vi "FTW-Actor.vi"(0 "DD Actor Template-Core In":refnum<class "DD Actor Template-Core.lvclass">, 5 "FTW Actor Instance Configuration":string="{\n  \"Identity\": \"ActorName\",\n  \"InboxAddress\": \"inproc://*\",\n  \"LoggerAddress\": \"\",\n  \"My Data\": false,\n  \"Publisher URI\": \"inproc://*\",\n  \"Subscriber URIs\": \"\",\n  \"Refresh Period\": 2\n}", 11 "ErrorIn":errorcluster) -> (15 "Error":errorcluster)   [LabVIEW 2018, in "DD Actor Template-Core.lvclass"]
uses:
  DD Actor Template-Core.lvclass
  C:/Jobs/Featherweight/featherweight-2018/source/actor/Instance/FTW-ActorInstance.lvclass
  DD Actor Template-Core.lvclass/DD Actor Template-Core.ctl
  source/actor/Instance/FTW-ActorInstance.lvclass/FTW-ActorInstance.ctl
  b528c082-742f-4d18-8b03-c390aae6fd68.vi
  b528c082-742f-4d18-8b03-c390aae6fd68.vi/37bc4ba9-e295-41d8-9da2-04944fffb029.vi
  source/container/FTW-Container-FromVariant.vi
  source/container/FTW-Container-New-FromContainer.vi
  source/JSON/FTW-JSON-SerializeAndDestroy.vi
  source/actor/JobSequencer/FTW-SEQ-Current.vi
  source/actor/Message/Base/FTW-Message.lvclass
  source/actor/Connector/FTW-ActorConnector.lvclass
  source/actor/Instance/FTW-ActorInstance.lvclass
  source/actor/Message/Request/FTW-Message-IncomingRequest.lvclass
  source/actor/Publisher/FTW-Publisher.lvclass
  source/actor/Subscriber/FTW-Subscriber.lvclass
panel:
  # "#TODO\nhide controls for a GUI"
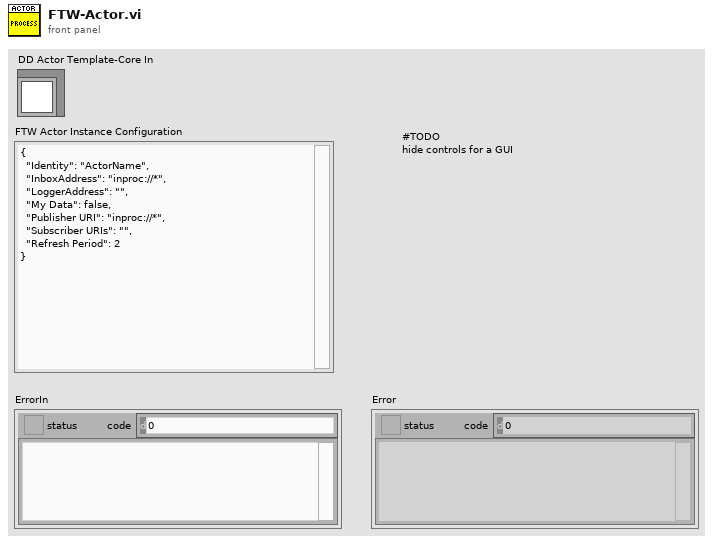
[diagram p1: front panel]
types:
  T1 = cluster{"Incoming Requests":refnum<event-registration>, "Local Messages":refnum<event-registration>, "Subscriber Registration":refnum<event-registration>}
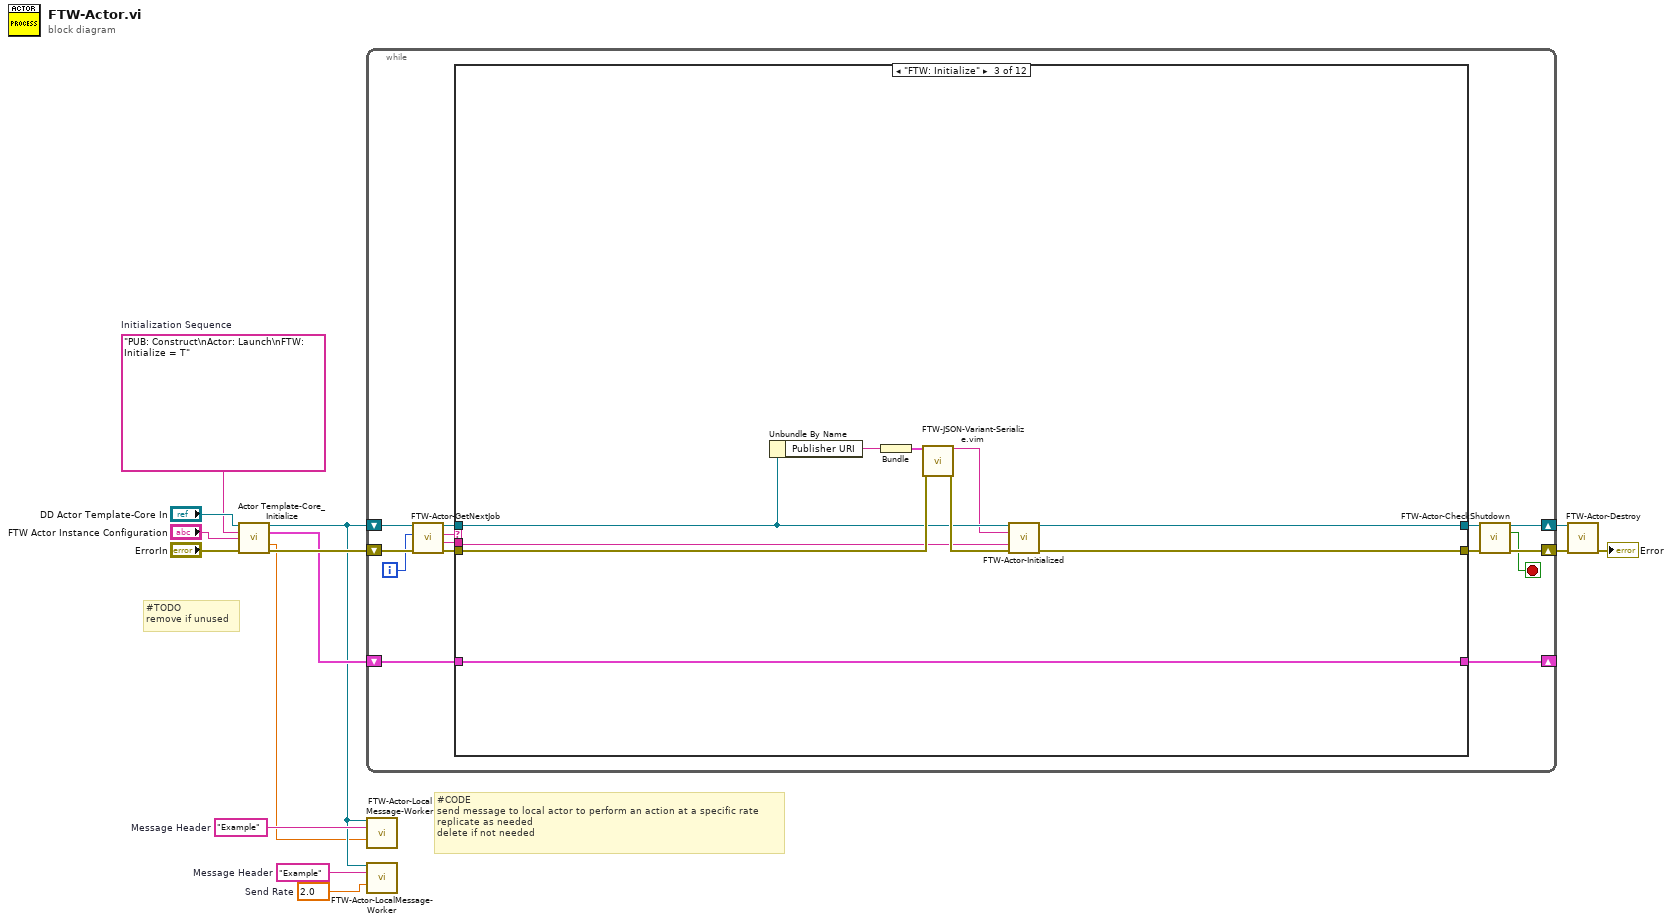
[diagram p0: block diagram]
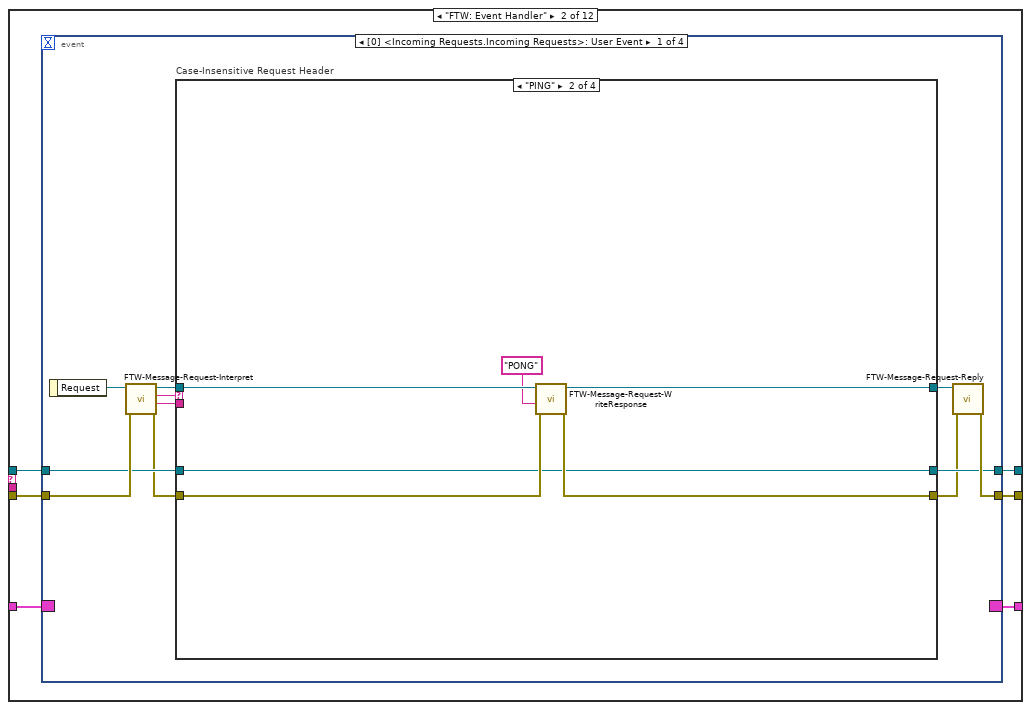
[diagram p3: hidden frame]
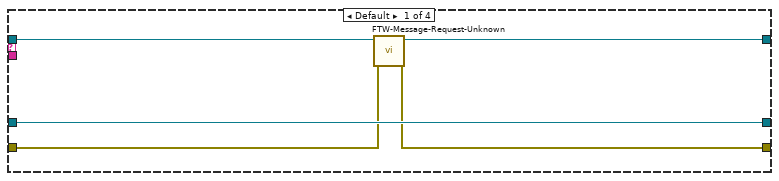
[diagram p4: hidden frame]
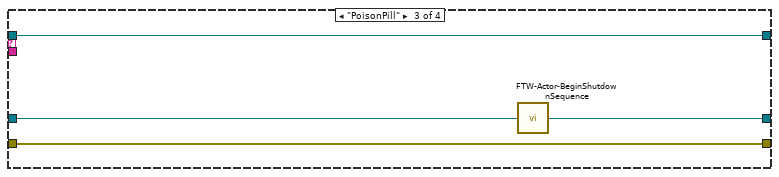
[diagram p5: hidden frame]
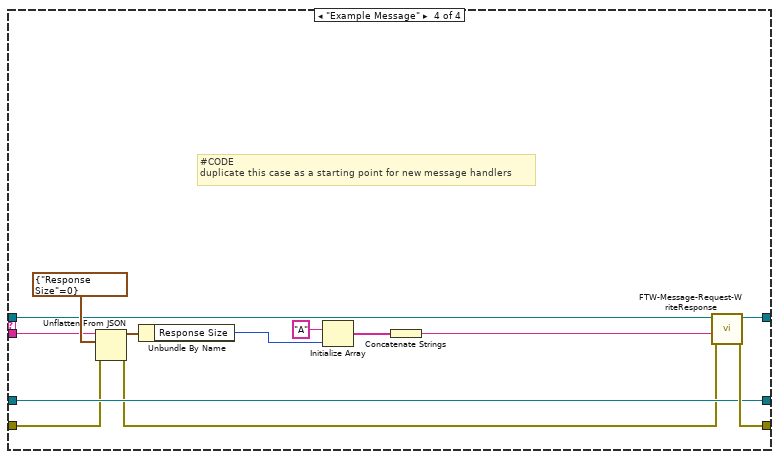
[diagram p6: hidden frame]
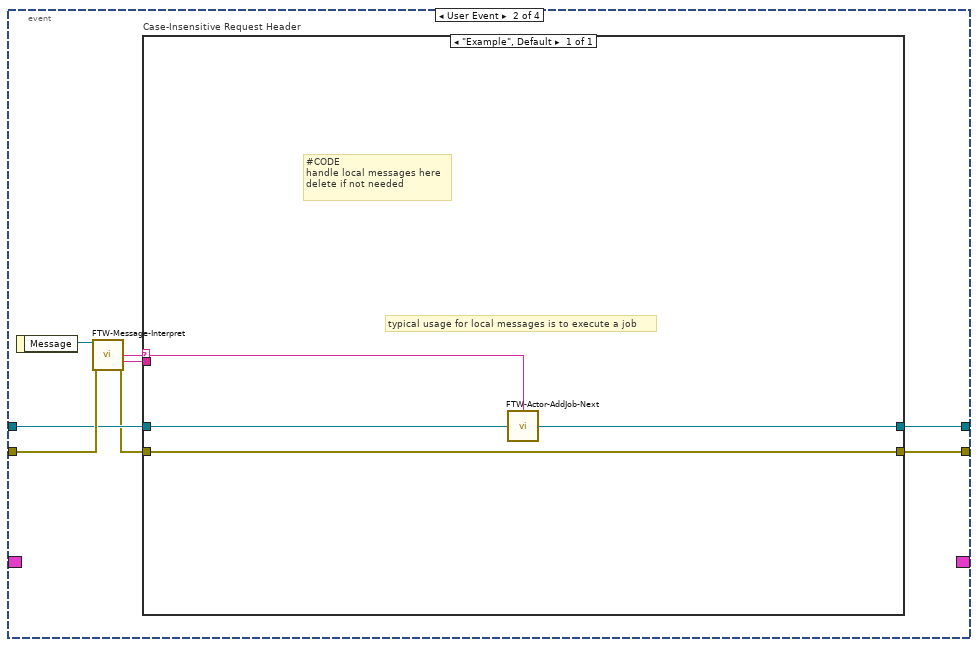
[diagram p7: hidden frame]
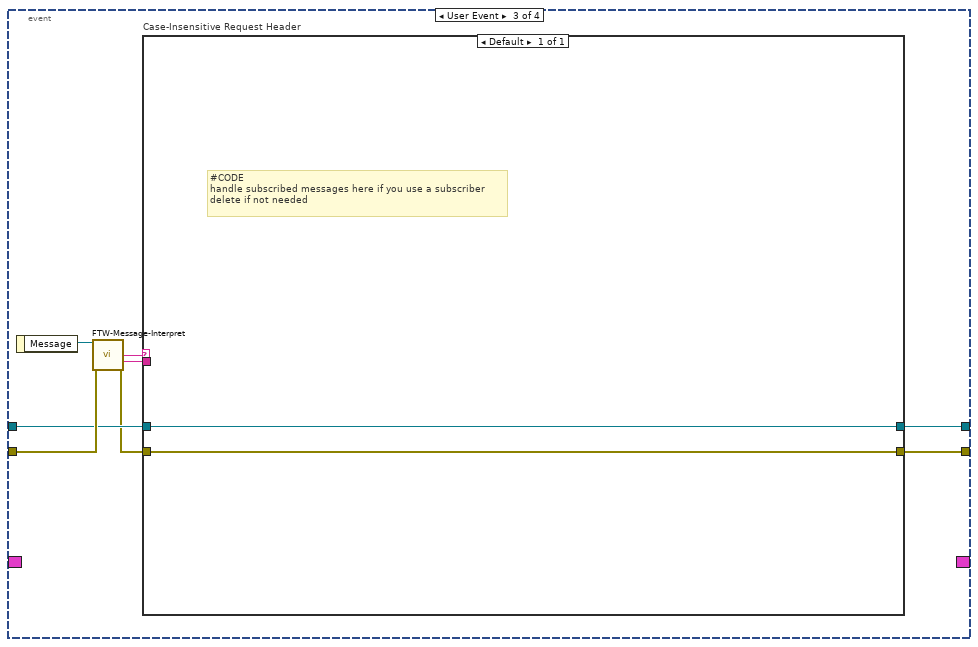
[diagram p8: hidden frame]
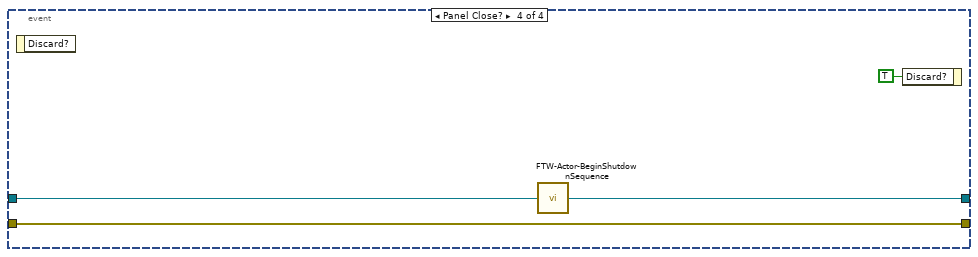
[diagram p9: hidden frame]
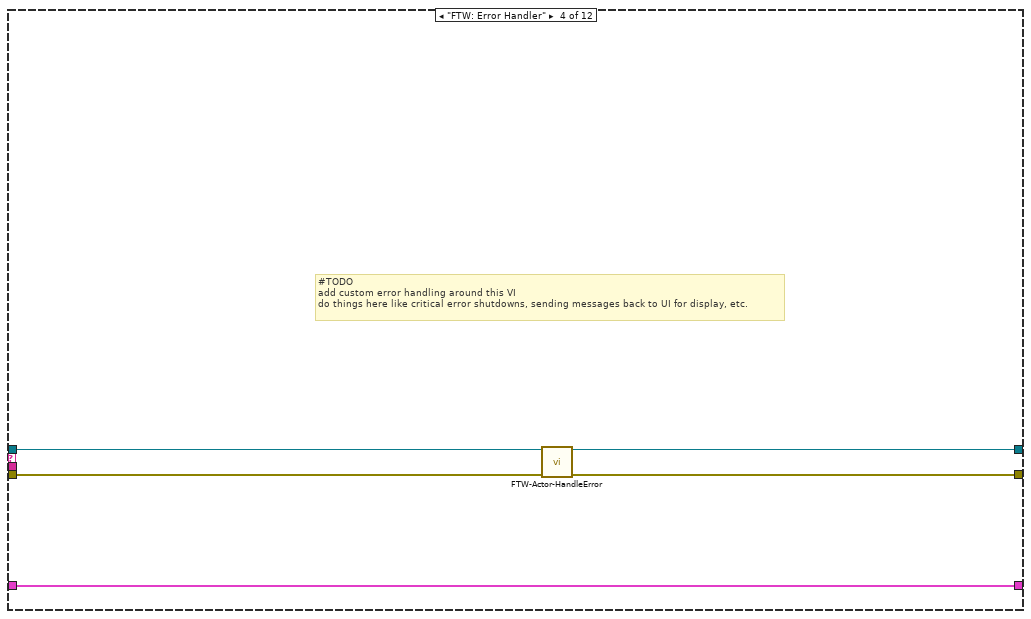
[diagram p10: hidden frame]
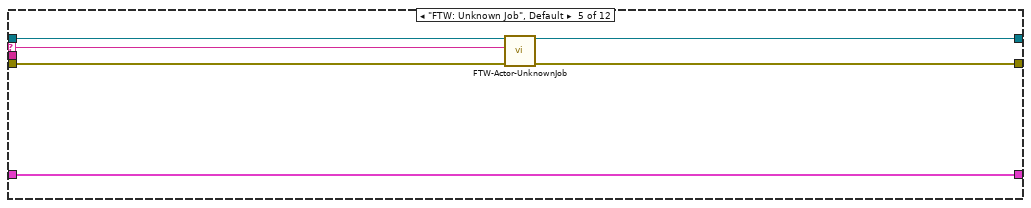
[diagram p11: hidden frame]
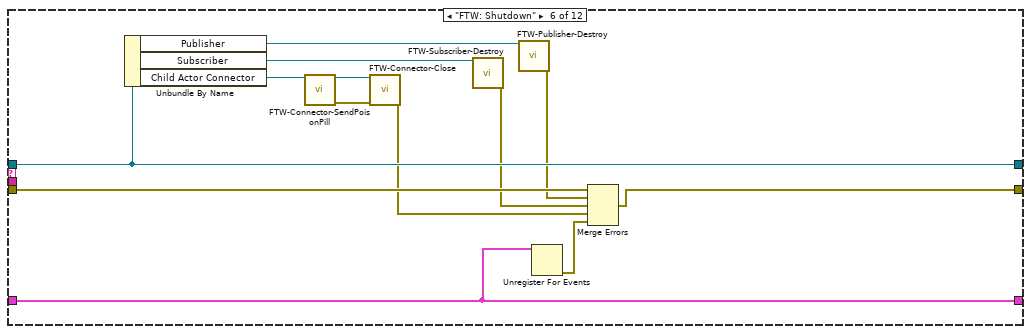
[diagram p12: hidden frame]
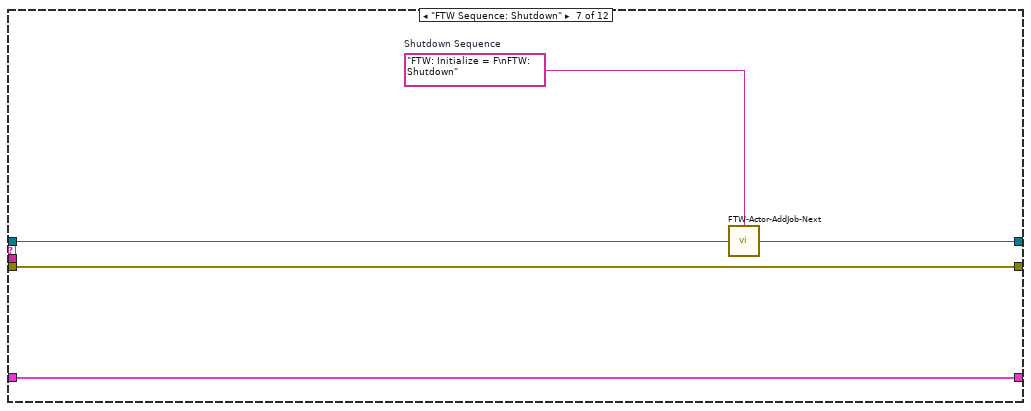
[diagram p13: hidden frame]
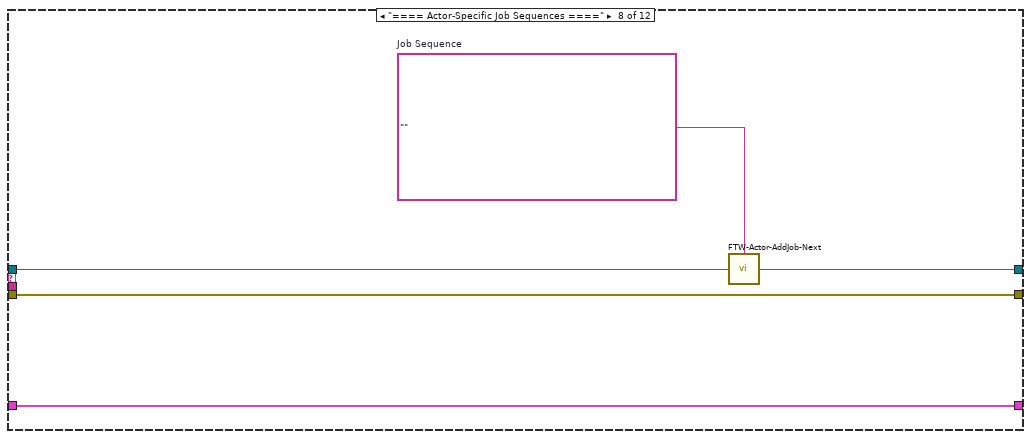
[diagram p14: hidden frame]
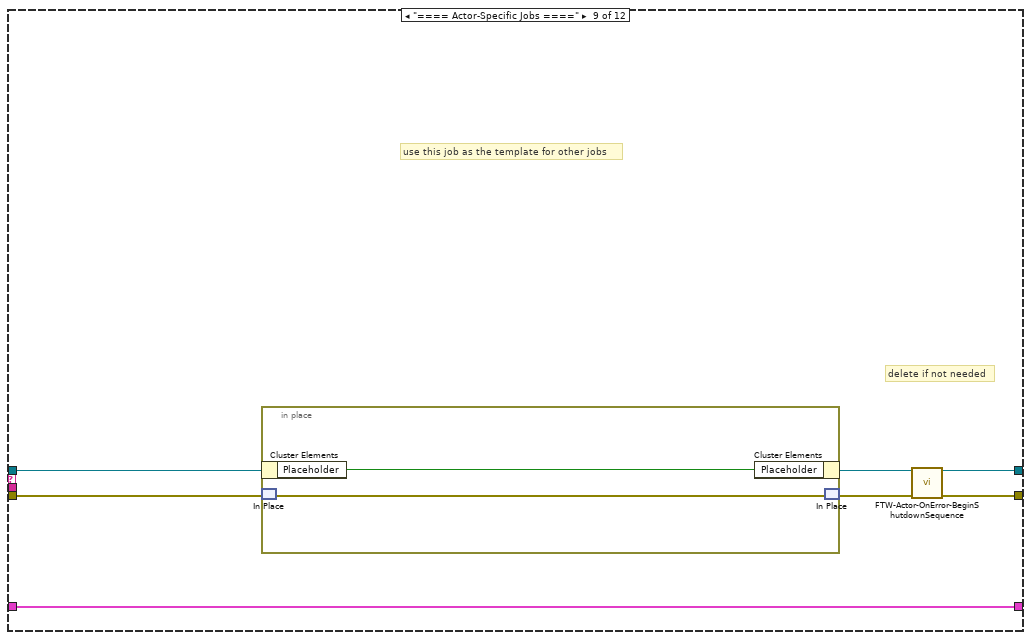
[diagram p15: hidden frame]
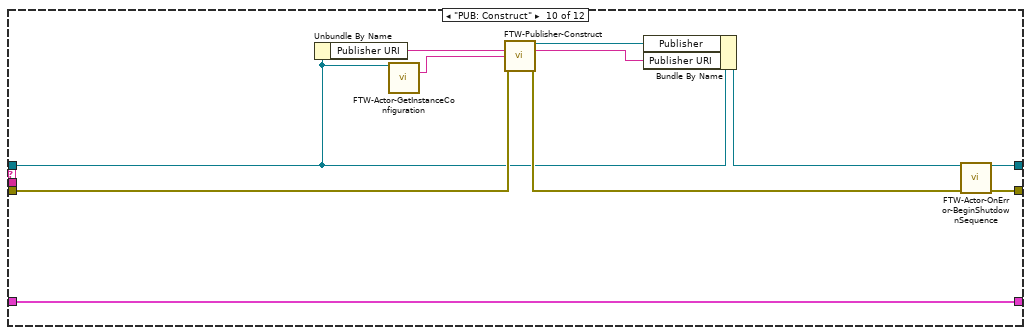
[diagram p16: hidden frame]
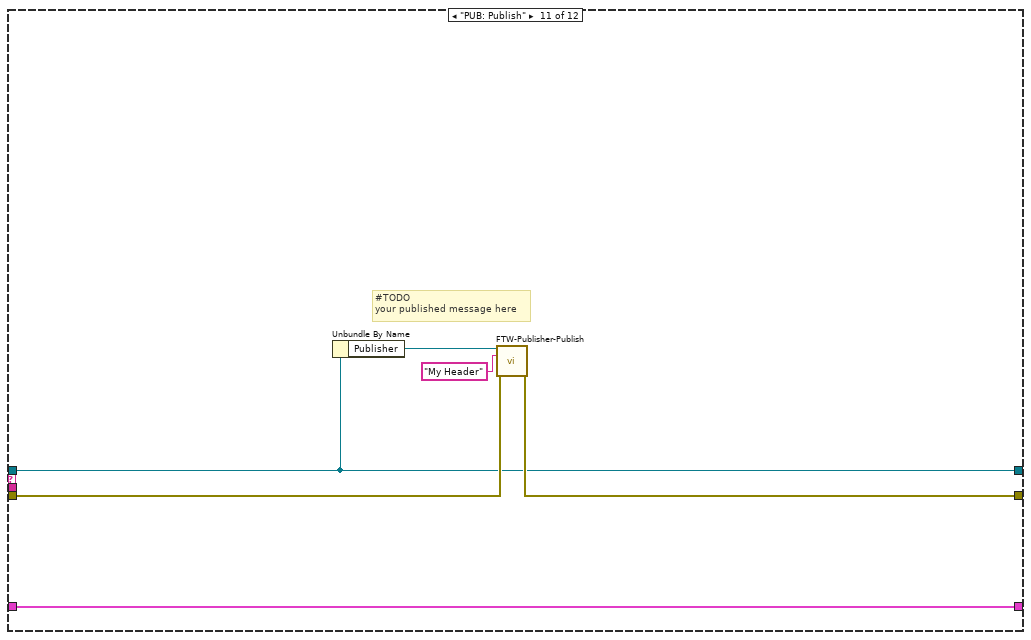
[diagram p17: hidden frame]
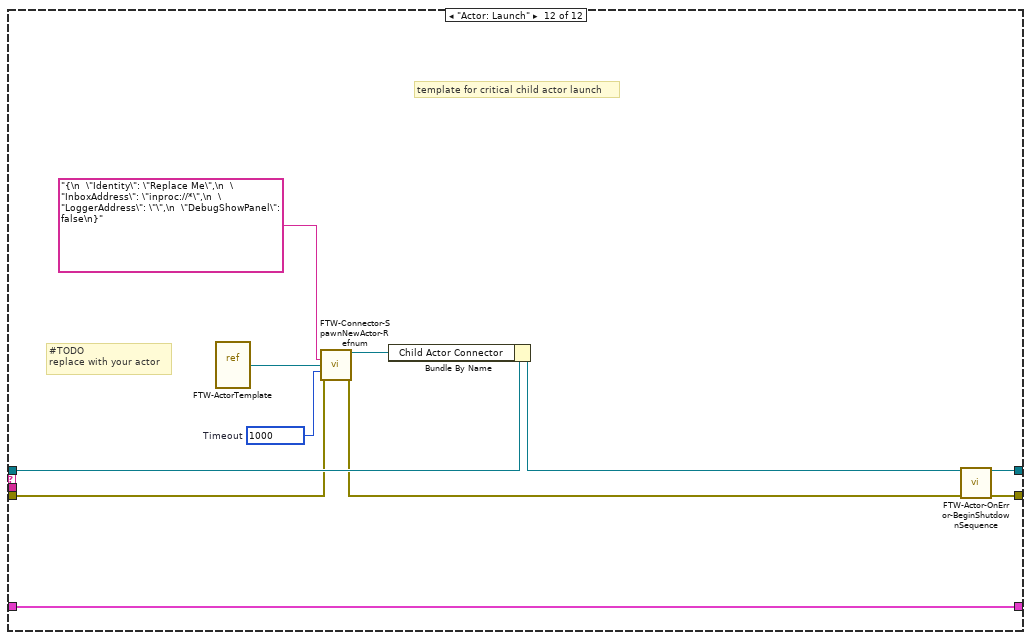
[diagram p18: hidden frame]
diagram:
  w7 = 2.0  # Send Rate
  w6 = "Example"  # Message Header
  w8 = "Example"  # Message Header
  w1 = "PUB: Construct\nActor: Launch\nFTW: Initialize = T"  # Initialization Sequence
  # "#CODE\nsend message to local actor to perform an action at a specific rate\nreplicate as needed\ndelete if not needed"
  # "#TODO\nremove if unused"
  n1 = call "Actor Template-Core_Initialize.vi"("DD Actor Template-Core In"="DD Actor Template-Core In", "Initialization Sequence"=w1, "FTW Actor Instance Configuration"="FTW Actor Instance Configuration", "error in (no error)"="ErrorIn") -> ("DD Actor Template-Core Out"=w5:refnum<class "DD Actor Template-Core.lvclass">, "Event Refnums"=w9:T1, "Refresh Period"=w4:dbl, "error out"=w11:errorcluster)  [unwired: 8 in]
  n2 = while {
    shift-right: [w18] -> w13
    shift-left: w11 -> [w25]
    shift-right: [w15] -> _
    shift-left: w9 -> [w28]
    shift-right: [w20] -> w14
    shift-left: w5 -> [w27]
    i -> [w16]
    stop <- w17 stop-if-true
    n3 = call "FTW-Actor-GetNextJob.vi"("error in"=w25, "Jobs Performed"=w16, "FTW Actor Instance"=w27) -> ("error out"=w24:errorcluster, "Job Data"=w22:string, "Job Name"=w23:string, "FTW Actor Instance out"=w26:refnum<class "DD Actor Template-Core.lvclass">)  [unwired: 5 in]
    n4 = case shown="\"FTW: Initialize\"" w23 {
      selector: w23 -> [_ _ _ _ w118 _ _ _ _ _ _ _]
      tunnel: [w30 w37 w108 w113 w121 w135 w140 w145 w149 w162 w170 w182] -> w19
      tunnel: w24 -> [w30 w36 w112 w115 w122 w136 w140 w145 w152 w164 w171 w176]
      tunnel: w28 -> [w31 w32 w110 w117 w123 w133 w141 w146 w153 w166 w172 w183]
      tunnel: [w31 w35 w110 w117 w123 w133 w141 w146 w153 w166 w172 w183] -> w15
      tunnel: w22 -> [_ _ w105 _ _ _ _ _ _ _ _ _]
      tunnel: [w29 w34 w109 w114 w119 w132 w138 w143 w147 w160 w169 w181] -> w21
      tunnel: w26 -> [w29 w33 w107 w116 w120 w132 w139 w144 w150 w157 w169 w180]
      frame "==== Featherweight Framework Jobs ====" {
      }
      frame "FTW: Event Handler" {
        n5 = event shown="[0] <Incoming Requests.Incoming Requests>: User Event" {
          selector: w32 -> [_ _ _ _]
          dyn-events: [_ _ _ _] -> w35
          timeout: _ -> [_ _ _ _]
          tunnel: [w47 w79 w91 w101] -> w37
          tunnel: w36 -> [w46 w83 w95 w101]
          tunnel: [w41 w80 w92 w99] -> w34
          tunnel: w33 -> [w45 w82 w94 w100]
          event User Event {
            n6 = event-data() -> ("Request"=w48:refnum<class "FTW-Message-IncomingRequest.lvclass">)  [unwired: 1 in]
            n7 = call "FTW-Message-Request-Interpret.vi"("error in"=w46, "FTW Incoming Request"=w48) -> ("error out"=w44:errorcluster, "Request Body"=w38:string, "Request Header"=w42:string, "FTW Incoming Request out"=w43:refnum<class "FTW-Message-IncomingRequest.lvclass">)  [unwired: 6 in]
            n8 = case "Case-Insensitive Request Header" shown="\"PING\"" w42 {
              tunnel: [w51 w57 w62 w76] -> w40
              tunnel: w44 -> [w52 w58 w62 w65]
              tunnel: [w53 w56 w63 w74] -> w41
              tunnel: w45 -> [w53 w56 w61 w74]
              tunnel: w43 -> [w50 w59 w60 w66]
              tunnel: [w49 w55 w60 w75] -> w39
              tunnel: w38 -> [_ _ _ w64]
              frame Default {
                n9 = call "FTW-Message-Request-Unknown.vi"("error in"=w52, "FTW Incoming Request"=w50) -> ("error out"=w51:errorcluster, "FTW Incoming Request Out"=w49:refnum<class "FTW-Message-IncomingRequest.lvclass">)  [unwired: 8 in]
              }
              frame "PING" {
                n10 = call "FTW-Message-Request-WriteResponse.vi"("error in"=w58, "Response Body"="PONG" ("Response Header"), "FTW Incoming Request"=w59) -> ("error out"=w57:errorcluster, "FTW Incoming Request out"=w55:refnum<class "FTW-Message-IncomingRequest.lvclass">)  [unwired: 7 in]
              }
              frame "PoisonPill" {
                n11 = call "FTW-Actor-BeginShutdownSequence.vi"("FTW Actor Instance"=w61) -> ("FTW Actor Instance out"=w63:refnum<class "DD Actor Template-Core.lvclass">)  [unwired: 3 in]
              }
              frame "Example Message" {
                # "#CODE\nduplicate this case as a starting point for new message handlers"
                n12 = Unflatten From JSON(JSON string=w64, type and defaults=cluster{"Response Size":i32} {"Response Size"=0}, error in (no error)=w65) -> (value=w71:cluster{"Response Size":i32}, error out=w73:errorcluster)  [unwired: 4 in]
                n13 = Unbundle By Name(w71) -> ("Response Size"=w70:i32)
                n14 = Initialize Array("A", w70) -> (w68:string[])
                n15 = Concatenate Strings(w68) -> (w67:string)
                n16 = call "FTW-Message-Request-WriteResponse.vi"("error in"=w73, "Response Body"=w67, "FTW Incoming Request"=w66) -> ("error out"=w76:errorcluster, "FTW Incoming Request out"=w75:refnum<class "FTW-Message-IncomingRequest.lvclass">)  [unwired: 7 in]
              }
            }
            n17 = call "FTW-Message-Request-Reply.vi"("FTW: Reply Error"=w40, "FTW Incoming Request"=w39) -> ("error out"=w47:errorcluster)  [unwired: 8 in, 1 out]
          }
          event User Event {
            n18 = event-data() -> ("Message"=w84:refnum<class "FTW-Message.lvclass">)  [unwired: 1 in]
            n19 = call-dynamic "FTW-Message-Interpret.vi"("FTW Message"=w84, "error in"=w83) -> ("Message Header"=w78:string, "Message Body"=w77:string, "error out"=w81:errorcluster)  [unwired: 9 in, 2 out]
            n20 = case "Case-Insensitive Request Header" shown="\"Example\", Default" w78 {
              selector: w78 -> [w85]
              tunnel: [w87] -> w79
              tunnel: w81 -> [w87]
              tunnel: [w86] -> w80
              tunnel: w82 -> [w88]
              tunnel: w77 -> [_]
              frame "Example", Default {
                # "#CODE\nhandle local messages here\ndelete if not needed"
                # "typical usage for local messages is to execute a job"
                n21 = call "FTW-Actor-AddJob-Next.vi"("Add Next in Job Queue"=w85, "FTW Actor Instance"=w88) -> ("FTW Actor Instance out"=w86:refnum<class "DD Actor Template-Core.lvclass">)  [unwired: 2 in]
              }
            }
          }
          event User Event {
            n22 = event-data() -> ("Message"=w96:refnum<class "FTW-Message.lvclass">)  [unwired: 1 in]
            n23 = call-dynamic "FTW-Message-Interpret.vi"("FTW Message"=w96, "error in"=w95) -> ("Message Header"=w90:string, "Message Body"=w89:string, "error out"=w93:errorcluster)  [unwired: 9 in, 2 out]
            n24 = case "Case-Insensitive Request Header" shown="Default" w90 {
              tunnel: [w97] -> w91
              tunnel: w93 -> [w97]
              tunnel: [w98] -> w92
              tunnel: w94 -> [w98]
              tunnel: w89 -> [_]
              frame Default {
                # "#CODE\nhandle subscribed messages here if you use a subscriber\ndelete if not needed"
              }
            }
          }
          event Panel Close? {
            n25 = event-data() -> ()  [unwired: 1 in, 1 out]
            n26 = call "FTW-Actor-BeginShutdownSequence.vi"("FTW Actor Instance"=w100) -> ("FTW Actor Instance out"=w99:refnum<class "DD Actor Template-Core.lvclass">)  [unwired: 3 in]
            n27 = event-data("Discard?"=TRUE) -> ()  [unwired: 1 in, 1 out]
          }
        }
      }
      frame "FTW: Initialize" {
        n28 = Unbundle By Name(w107) -> ("Publisher URI"=w106:string)
        n29 = Bundle("Publisher URI"=w106) -> (w104:cluster{"Publisher URI":string})  [unwired: 1 in]
        n30 = call "FTW-JSON-Variant-Serialize.vim"("Variant"=w104, "error in"=w112) -> ("JSON String"=w103:string, "error out"=w111:errorcluster)  [unwired: 12 in]
        n31 = call-dynamic "FTW-Actor-Initialized.vi"("FTW Actor Instance"=w107, "Initialized Response"=w103, "Positive Init?"=w105, "error in"=w111) -> ("FTW Actor Instance out"=w109:refnum<class "DD Actor Template-Core.lvclass">, "error out"=w108:errorcluster)  [unwired: 10 in]
      }
      frame "FTW: Error Handler" {
        # "#TODO\nadd custom error handling around this VI\ndo things here like critical error shutdowns, sending messages back to UI for display, etc."
        n32 = call-dynamic "FTW-Actor-HandleError.vi"("FTW Actor Instance"=w116, "error in"=w115) -> ("FTW Actor Instance out"=w114:refnum<class "DD Actor Template-Core.lvclass">, "error out"=w113:errorcluster)  [unwired: 10 in, 2 out]
      }
      frame "FTW: Unknown Job", Default {
        n33 = call-dynamic "FTW-Actor-UnknownJob.vi"("FTW Actor Instance"=w120, "Unknown Job"=w118, "error in"=w122) -> ("FTW Actor Instance out"=w119:refnum<class "DD Actor Template-Core.lvclass">, "error out"=w121:errorcluster)  [unwired: 11 in]
      }
      frame "FTW: Shutdown" {
        n34 = Unbundle By Name(w132) -> ("Publisher"=w131:refnum<class "FTW-Publisher.lvclass">, "Subscriber"=w129:refnum<class "FTW-Subscriber.lvclass">, "Child Actor Connector"=w127:refnum<class "FTW-ActorConnector.lvclass">)
        n35 = call-dynamic "FTW-Connector-SendPoisonPill.vi"("FTW Actor Connector"=w127) -> ("FTW Actor Connector out"=w126:refnum<class "FTW-ActorConnector.lvclass">, "error out"=w125:errorcluster)  [unwired: 9 in, 4 out]
        n36 = call-dynamic "FTW-Connector-Close.vi"("FTW Actor Connector"=w126, "error in"=w125) -> ("error out"=w124:errorcluster)  [unwired: 13 in]
        n37 = call "FTW-Subscriber-Destroy.vi"("FTW-Subscription In"=w129) -> ("error out"=w128:errorcluster)  [unwired: 14 in]
        n38 = call "FTW-Publisher-Destroy.vi"("FTW-Publisher In"=w131) -> ("error out"=w130:errorcluster)  [unwired: 14 in]
        n39 = Unregister For Events(event registration refnum=w133) -> (error out=w134:errorcluster)  [unwired: 1 in]
        n40 = Merge Errors(w136, w130, w128, w124, w134) -> (w135:errorcluster)
      }
      frame "FTW Sequence: Shutdown" {
        w137 = "FTW: Initialize = F\nFTW: Shutdown"  # Shutdown Sequence
        n41 = call "FTW-Actor-AddJob-Next.vi"("Add Next in Job Queue"=w137, "FTW Actor Instance"=w139) -> ("FTW Actor Instance out"=w138:refnum<class "DD Actor Template-Core.lvclass">)  [unwired: 2 in]
      }
      frame "==== Actor-Specific Job Sequences ====" {
        w142 = ""  # Job Sequence
        n42 = call "FTW-Actor-AddJob-Next.vi"("Add Next in Job Queue"=w142, "FTW Actor Instance"=w144) -> ("FTW Actor Instance out"=w143:refnum<class "DD Actor Template-Core.lvclass">)  [unwired: 2 in]
      }
      frame "==== Actor-Specific Jobs ====" {
        # "delete if not needed"
        # "use this job as the template for other jobs"
        n43 = in-place {
          n44 = in-place-cluster #1(w150) -> ("Placeholder"=w154:bool)
          n45 = in-place-match #2(w152) -> (w155:errorcluster)
          n46 = in-place-cluster #1("Placeholder"=w154) -> (w148:refnum<class "DD Actor Template-Core.lvclass">)
          n47 = in-place-match #2(w155) -> (w151:errorcluster)
        }
        n48 = call-dynamic "FTW-Actor-OnError-BeginShutdownSequence.vi"("FTW Actor Instance"=w148, "error in"=w151) -> ("FTW Actor Instance out"=w147:refnum<class "DD Actor Template-Core.lvclass">, "error out"=w149:errorcluster)  [unwired: 12 in]
      }
      frame "PUB: Construct" {
        n49 = Unbundle By Name(w157) -> ("Publisher URI"=w158:string)
        n50 = call "FTW-Actor-GetInstanceConfiguration.vi"("FTW Actor Instance"=w157) -> ("Identity"=w156:string)  [unwired: 12 in, 2 out]
        n51 = call "FTW-Publisher-Construct.vi"("Address"=w158, "Identity"=w156, "error in"=w164) -> ("FTW-Publisher Out"=w165:refnum<class "FTW-Publisher.lvclass">, "Actual Address"=w159:string, "error out"=w163:errorcluster)  [unwired: 10 in]
        n52 = Bundle By Name(cluster=w157, "Publisher"=w165, "Publisher URI"=w159) -> (w161:refnum<class "DD Actor Template-Core.lvclass">)
        n53 = call-dynamic "FTW-Actor-OnError-BeginShutdownSequence.vi"("FTW Actor Instance"=w161, "error in"=w163) -> ("FTW Actor Instance out"=w160:refnum<class "DD Actor Template-Core.lvclass">, "error out"=w162:errorcluster)  [unwired: 12 in]
      }
      frame "PUB: Publish" {
        # "#TODO\nyour published message here"
        n54 = Unbundle By Name(w169) -> ("Publisher"=w168:refnum<class "FTW-Publisher.lvclass">)
        n55 = call "FTW-Publisher-Publish.vi"("FTW-Publisher In"=w168, "Header"="My Header", "error in"=w171) -> ("error out"=w170:errorcluster)  [unwired: 11 in, 1 out]
      }
      frame "Actor: Launch" {
        w179 = 1000  # Timeout
        # "#TODO\nreplace with your actor"
        # "template for critical child actor launch"
        n56 = vi-ref "FTW-ActorTemplate.vi"() -> (w178:refnum<vi>)
        n57 = call "FTW-Connector-SpawnNewActor-Refnum.vi"("Configuration"="{\n  \"Identity\": \"Replace Me\",\n  \"InboxAddress\": \"inproc://*\",\n  \"LoggerAddress\": \"\",\n  \"DebugShowPanel\": false\n}", "Actor VI Refnum"=w178, "Timeout"=w179, "error in"=w176) -> ("FTW Actor Connector"=w173:refnum<class "FTW-ActorConnector.lvclass">, "error out"=w175:errorcluster)  [unwired: 8 in, 2 out]
        n58 = Bundle By Name(cluster=w180, "Child Actor Connector"=w173) -> (w174:refnum<class "DD Actor Template-Core.lvclass">)
        n59 = call-dynamic "FTW-Actor-OnError-BeginShutdownSequence.vi"("FTW Actor Instance"=w174, "error in"=w175) -> ("FTW Actor Instance out"=w181:refnum<class "DD Actor Template-Core.lvclass">, "error out"=w182:errorcluster)  [unwired: 12 in]
      }
    }
    n60 = call "FTW-Actor-CheckShutdown.vi"("FTW Actor Instance"=w21, "error in"=w19) -> ("FTW Actor Instance out"=w20:refnum<class "DD Actor Template-Core.lvclass">, "Shutdown?"=w17:bool, "error out"=w18:errorcluster)  [unwired: 11 in]
  }
  n61 = call "FTW-Actor-LocalMessage-Worker.vi"("FTW-ActorInstance In"=w5, "Message Header"=w8, "Send Rate"=w4) -> ()  [unwired: 13 in]
  n62 = call "FTW-Actor-LocalMessage-Worker.vi"("FTW-ActorInstance In"=w5, "Message Header"=w6, "Send Rate"=w7) -> ()  [unwired: 13 in]
  n63 = call-dynamic "FTW-Actor-Destroy.vi"("FTW Actor Instance"=w14, "error in"=w13) -> ("error out"=→"Error":errorcluster)  [unwired: 13 in]
